vi "FPServer.vi"(0 "reference in":refnum<class "FrontPanelManager.lvclass">, 5 "error in":errorcluster) -> (14 "reference out":refnum<class "FrontPanelManager.lvclass">, 19 "error out":errorcluster)   [LabVIEW 2014, in "FrontPanelPublisher.lvlib" / "FrontPanelManager.lvclass"]
uses:
  FrontPanelManager.lvclass
  WebFrontPanel_class/WebFrontPanel.lvclass
  Websocket_class/Websocket.lvclass
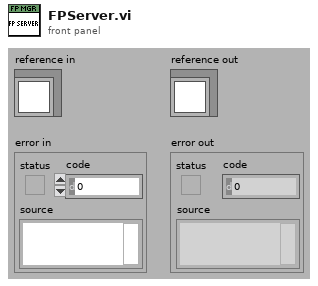
[diagram p1: front panel]
types:
  T1 = typedef "FrontPanelPublisher.lvlib/FrontPanelManager.lvclass/FPServerMessage.ctl" = cluster{"Message":string, "Page":string, "Data":string[][], "Connection ID":u64}
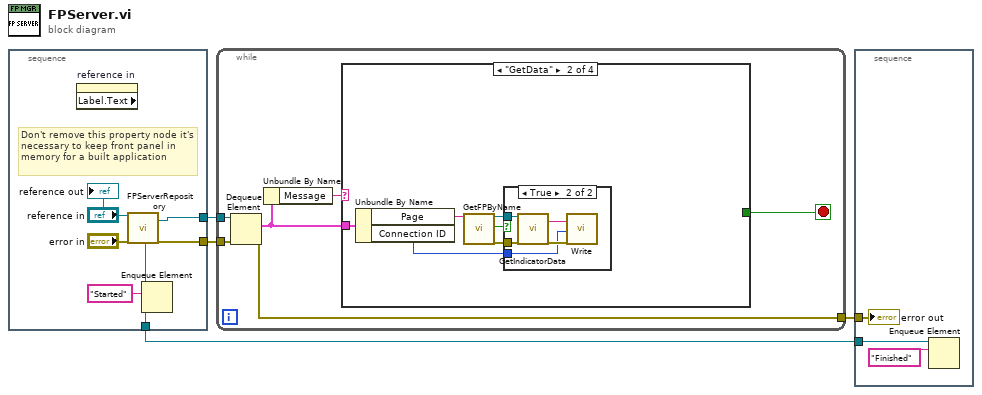
[diagram p0: block diagram]
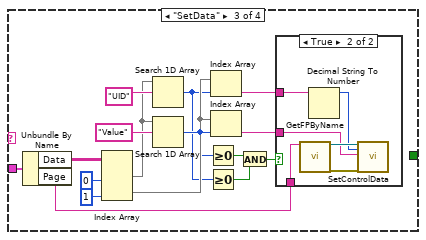
[diagram p4: hidden frame]
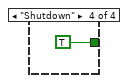
[diagram p6: hidden frame]
diagram:
  n1 = stacked-sequence {
    tunnel: [w8] -> w4
    tunnel: [w7] -> w2
    tunnel: [w5] -> w1
    frame #0 {
      # "Don't remove this property node it's necessary to keep front panel in memory for a built application"
      n2 = property on="reference in" class="LVClassControl (strict)" props=["Label", "Text"]() -> ()  [unwired: 2 in, 3 out]
      n3 = call "FPServerRepository.vi"("reference in"="reference in", "error in (no error)"="error in") -> ("ProcessSyncQueue"=w7:refnum<queue>, "ToProcessQueue"=w5:refnum<queue>, "error out"=w8:errorcluster)  [unwired: 11 in, 4 out]
      n4 = Enqueue Element(queue=w7, element="Started") -> ()  [unwired: 2 in, 3 out]
      "reference out" <- "reference in"
    }
  }
  n5 = while {
    tunnel: w1 -> [w16]
    tunnel: [w13] -> w3
    tunnel: w4 -> [w12]
    stop <- w14 stop-if-true
    n6 = Dequeue Element(queue=w16, error in (no error)=w12) -> (element=w11:T1, error out=w13:errorcluster)  [unwired: 1 in, 2 out]
    n7 = Unbundle By Name(w11) -> ("Message"=w15:string)
    n8 = case shown="\"GetData\"" w15 {
      tunnel: [_ _ _ TRUE] -> w14
      tunnel: w11 -> [_ w19 w28 _]
      frame Default {
      }
      frame "GetData" {
        n9 = Unbundle By Name(w19) -> ("Page"=w17:string, "Connection ID"=w18:u64)
        n10 = call "GetFPByName.vi"("WFP Name"=w17) -> ("WebFrontPanel"=w22:refnum<class "WebFrontPanel.lvclass">, "Found"=w20:bool, "error out"=w21:errorcluster)  [unwired: 16 in]
        n11 = case shown="True" w20 {
          tunnel: w22 -> [_ w27]
          tunnel: w21 -> [_ w26]
          tunnel: w18 -> [_ w23]
          frame False {
          }
          frame True {
            n12 = call-dynamic "GetIndicatorData.vi"("reference in"=w27, "error in (no error)"=w26) -> ("String"=w25:string, "error out"=w24:errorcluster)  [unwired: 15 in, 1 out]
            n13 = call "Write.vi"("Payload"=w25, "Connection ID"=w23, "error in"=w24) -> ()  [unwired: 15 in, 2 out]
          }
        }
      }
      frame "SetData" {
        n14 = Unbundle By Name(w28) -> ("Data"=w29:string[][], "Page"=w30:string)
        n15 = Index Array(array=w29, index (col) #1=0 ("disabled index (col)"), index (col) #2=1 ("index (col)")) -> (element #1=w41:string[], element #2=w40:string[])  [unwired: 2 in]
        n16 = Search 1D Array(1D array=w41, element="UID") -> (index of element=w36:i32)  [unwired: 1 in]
        n17 = Search 1D Array(1D array=w41, element="Value") -> (index of element=w37:i32)  [unwired: 1 in]
        n18 = Greater Or Equal To 0?(x=w37) -> (x >= 0?=w35:bool)
        n19 = Greater Or Equal To 0?(x=w36) -> (x >= 0?=w34:bool)
        n20 = Index Array(array=w40, index=w36) -> (element=w39:string)
        n21 = Index Array(array=w40, index=w37) -> (element=w38:string)
        n22 = And(x=w35, y=w34) -> (x .and. y?=w33:bool)
        n23 = case shown="True" w33 {
          tunnel: w39 -> [_ w46]
          tunnel: w38 -> [_ w45]
          tunnel: w30 -> [_ w44]
          frame False {
          }
          frame True {
            n24 = call "GetFPByName.vi"("WFP Name"=w44) -> ("WebFrontPanel"=w49:refnum<class "WebFrontPanel.lvclass">, "error out"=w47:errorcluster)  [unwired: 16 in, 1 out]
            n25 = Decimal String To Number(string=w46) -> (number=w48:i32)  [unwired: 2 in, 1 out]
            n26 = call-dynamic "SetControlData.vi"("reference in"=w49, "UID"=w48, "Value"=w45, "error in (no error)"=w47) -> ()  [unwired: 14 in, 2 out]
          }
        }
      }
      frame "Shutdown" {
      }
    }
  }
  n27 = stacked-sequence {
    tunnel: w3 -> [w53]
    tunnel: w2 -> [w52]
    frame #0 {
      n28 = Enqueue Element(queue=w52, element="Finished") -> ()  [unwired: 2 in, 3 out]
      "error out" <- w53
    }
  }
